vi "Actual_step.vi"() -> ()   [LabVIEW 2017]
panel:
  out "Actual_step":dbl
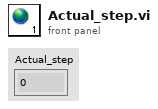
[diagram p1: front panel]
diagram:
